vi "FMSweep-Create (cluster).vi"(8 "error in (no error)":errorcluster, 9 "Npts":i32, 10 "Sampling Rate (Hz)":dbl, 11 "FMSweep In":T1) -> (0 "error out":errorcluster, 2 "Waveform":dbl[](array[numeric]), 3 "FMSweep Out":T1)   [LabVIEW 2020]
uses:
  FM Sweep Params.ctl
panel:
  out "Waveform Graph":dbl[](graph)
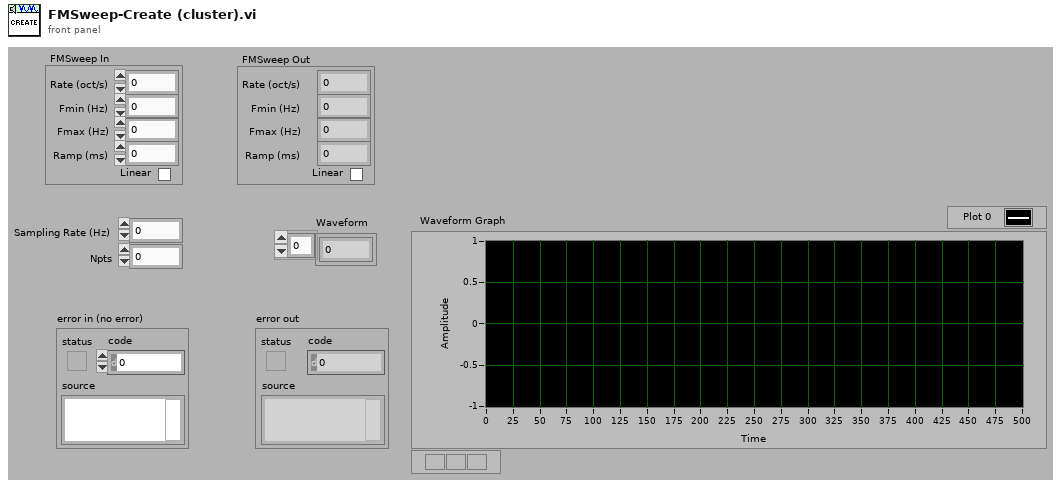
[diagram p1: front panel]
types:
  T1 = typedef "FM Sweep Params.ctl" = cluster{"Rate (oct/s)":dbl, "Fmin (Hz)":dbl, "Fmax (Hz)":dbl, "Ramp (ms)":dbl, "Linear":bool}
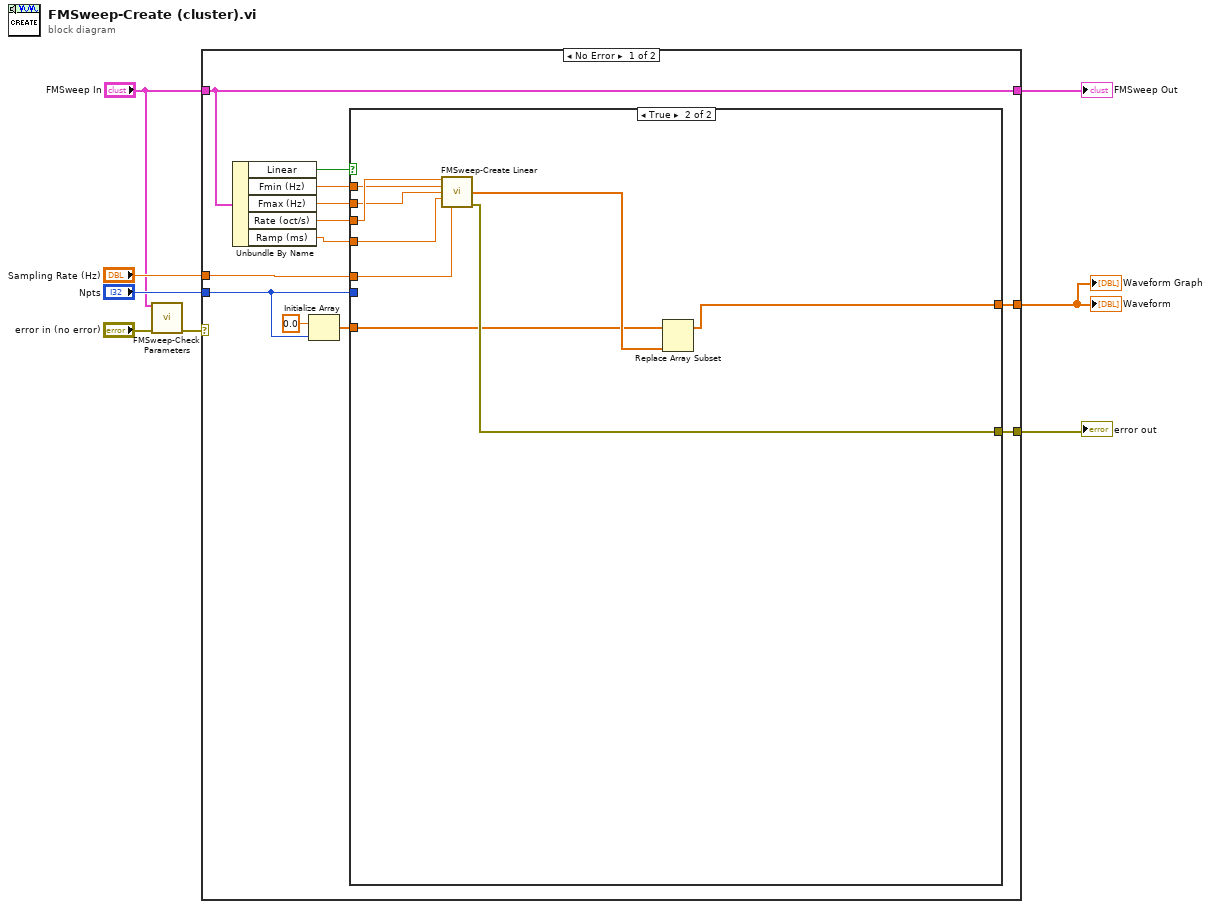
[diagram p0: block diagram]
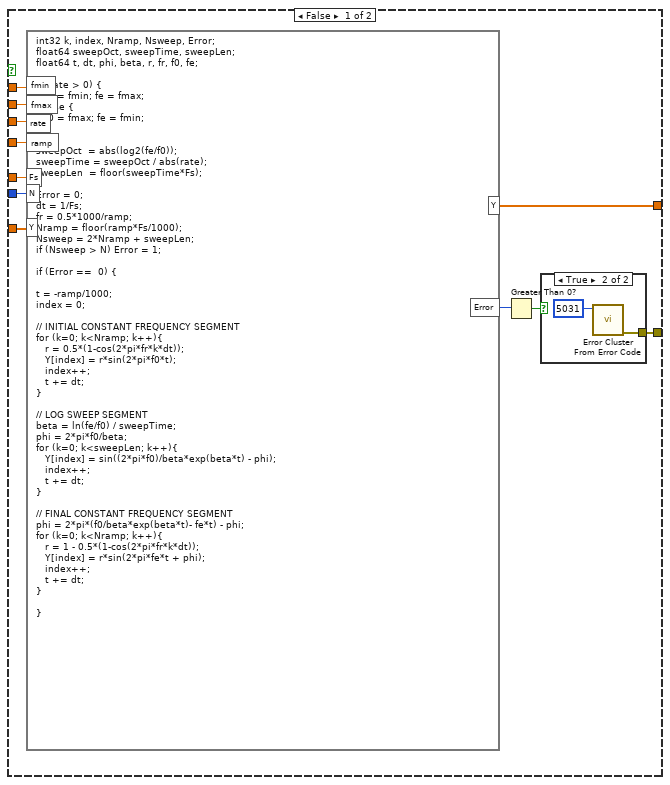
[diagram p2: hidden frame]
diagram:
  n1 = call "FMSweep-Check Parameters.vi"("FMSweep"="FMSweep In", "error in (no error)"="error in (no error)") -> ("error out"=w2:errorcluster)  [unwired: 13 in]
  n2 = case shown="No Error" w2 {
    selector: w2 -> [_ w44]
    tunnel: [w10 w44] -> w8
    tunnel: [w15 w43] -> w7
    tunnel: "FMSweep In" -> [w15 w43]
    tunnel: "Npts" -> [w13 _]
    tunnel: "Sampling Rate (Hz)" -> [w16 _]
    tunnel: [w14 _] -> w4
    frame No Error {
      n3 = Unbundle By Name(w15) -> ("Linear"=w9:bool, "Fmin (Hz)"=w20:dbl, "Fmax (Hz)"=w19:dbl, "Rate (oct/s)"=w18:dbl, "Ramp (ms)"=w17:dbl)
      n4 = Initialize Array(0.0 ("element"), w13) -> (w11:dbl[])
      n5 = case shown="True" w9 {
        tunnel: w20 -> [w31 w41]
        tunnel: w19 -> [w30 w40]
        tunnel: w18 -> [w29 w42]
        tunnel: w17 -> [w28 w39]
        tunnel: w16 -> [w27 w34]
        tunnel: [w26 w35] -> w14
        tunnel: w13 -> [w25 _]
        tunnel: w11 -> [w24 w36]
        tunnel: [w21 w38] -> w10
        frame False {
          n6 = formula code="int32 k, index, Nramp, Nsweep, Error;\nfloat64 sweepOct, sweepTime, sweepLen;\nfloat64 t, dt, phi, beta, r, fr, f0, fe;\n\nif (rate > 0) {\n   f0 = fmin; fe = fmax;\n} else {\n   f0 = fmax; fe = fmin;\n}\n\nsweepOct  = abs(log2(fe/f0));\nsweepTime = sweepOct / abs(rate);\nsweepLen  = floor(sweepTime*Fs);\n\nError = 0;\ndt = 1/Fs;\nfr = 0.5*1000/ramp;\nNramp = floor(ramp*Fs/1000);\nNsweep = 2*Nramp + sweepLen;\nif (Nsweep > N) Error = 1;  \n\nif (Error ==  0) {\n\nt = -ramp/1000;\nindex = 0;\n\n// INITIAL CONSTANT FREQUENCY SEGMENT\nfor (k=0; k<Nramp; k++){\n   r = 0.5*(1-cos(2*pi*fr*k*dt));\n   Y[index] = r*sin(2*pi*f0*t);  \n   index++;\n   t += dt;\n}\n\n// LOG SWEEP SEGMENT\nbeta = ln(fe/f0) / sweepTime;\nphi = 2*pi*f0/beta;\nfor (k=0; k<sweepLen; k++){\n   Y[index] = sin((2*pi*f0)/beta*exp(beta*t) - phi);\n   index++;\n   t += dt;\n}\n\n// FINAL CONSTANT FREQUENCY SEGMENT\nphi = 2*pi*(f0/beta*exp(beta*t)- fe*t) - phi;\nfor (k=0; k<Nramp; k++){\n   r = 1 - 0.5*(1-cos(2*pi*fr*k*dt));\n   Y[index] = r*sin(2*pi*fe*t + phi);\n   index++;\n   t += dt;\n}\n\n}"("fmin"=w31, "fmax"=w30, "rate"=w29, "ramp"=w28, "Fs"=w27, "N"=w25, "Y"=w24) -> ("Y"=w26:dbl[], "Error"=w23:i32)
          n7 = Greater Than 0?(x=w23) -> (x > 0?=w22:bool)
          n8 = case shown="True" w22 {
            tunnel: [_ w32] -> w21
            frame False {
            }
            frame True {
              n9 = call <vilib>:"Error Cluster From Error Code.vi"("error code (0)"=5031) -> ("error out"=w32:errorcluster)  [unwired: 8 in]
            }
          }
        }
        frame True {
          n10 = call "FMSweep-Create Linear.vi"("Sweep Rate (Hz/s)"=w42, "Fmin (Hz)"=w41, "Fmax (Hz)"=w40, "Ramp (ms)"=w39, "Fs (Hz)"=w34) -> ("Array"=w37:dbl[], "error out"=w38:errorcluster)  [unwired: 8 in, 1 out]
          n11 = Replace Array Subset(array=w36, new element=w37) -> (w35:dbl[])  [unwired: 1 in]
        }
      }
    }
    frame Error {
    }
  }
  "error out" <- w8
  "FMSweep Out" <- w7
  "Waveform" <- w4
  "Waveform Graph" <- w4
